vi "Save RT Sequence.vi"(8 "error in (no error)":errorcluster, 11 "RT Sequence Ref in":refnum<k24>) -> (0 "error out":errorcluster, 3 "RT Sequence Ref out":refnum<k24>)   [LabVIEW 2016, in "RT Sequence Creator API.lvlib"]
uses:
  RT Sequence Creator API.lvlib
  NationalInstruments.VeriStand.RealTimeSequenceDefinitionApi
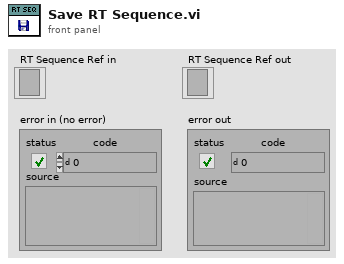
[diagram p1: front panel]
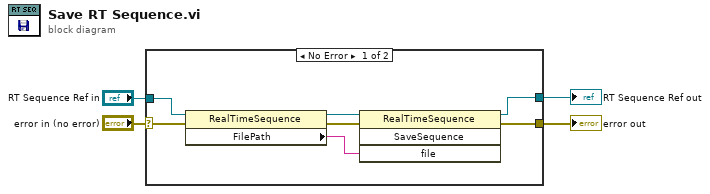
[diagram p0: block diagram]
diagram:
  n1 = case shown="No Error" "error in (no error)" {
    selector: "error in (no error)" -> [w11 w12]
    tunnel: "RT Sequence Ref in" -> [w7 w13]
    tunnel: [w10 w12] -> w2
    tunnel: [w9 w13] -> w1
    frame No Error {
      n2 = property class="RealTimeSequence"(reference=w7, error in=w11) -> (reference out=w6:refnum<k24>, error out=w8:errorcluster, "FilePath"=w5:string)
      n3 = invoke class="RealTimeSequence" method="SaveSequence"(reference=w6, error in=w8, "file"=w5) -> (reference out=w9:refnum<k24>, error out=w10:errorcluster)  [unwired: 1 in, 2 out]
    }
    frame Error {
    }
  }
  "RT Sequence Ref out" <- w1
  "error out" <- w2
